vi "Decimate Segments.vi"(5 "Y Buffer":dbl[](array[numeric]), 6 "Swap Axes":bool, 7 "X Buffer":dbl[](array[numeric]), 8 "px Lengths":i32[](array[numeric]), 9 "px Starts":i32[](array[numeric]), 10 "Independent":dbl[](array[numeric]), 11 "Dependent":dbl[](array[numeric])) -> (2 "Decimated Data":cluster{"X":dbl[], "Y":dbl[]})   [LabVIEW 2020, in "VolatusGUIElements.lvlib"]
uses:
  VolatusGUIElements.lvlib
panel:
  out "Last X":dbl format="%<%H:%M:%S%1u>T"
  out "First X":dbl format="%<%H:%M:%S%1u>T"
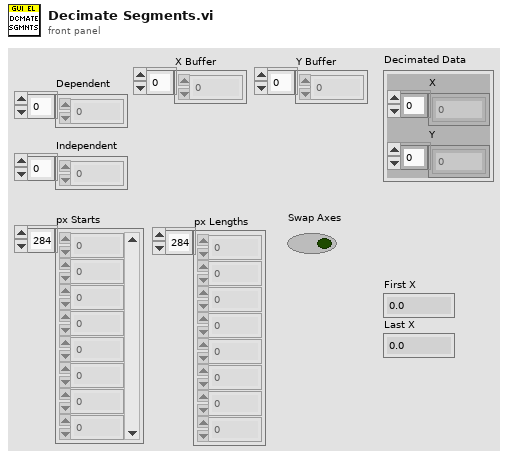
[diagram p1: front panel]
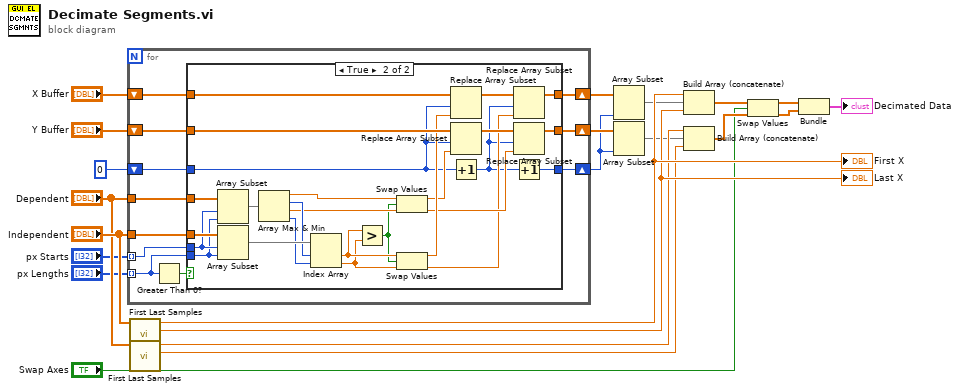
[diagram p0: block diagram]
diagram:
  n1 = for {
    shift-right: [w24] -> w11
    shift-left: "Y Buffer" -> [w27]
    shift-right: [w23] -> w12
    shift-left: "X Buffer" -> [w28]
    tunnel: "Independent" -> [w33]
    tunnel: "Dependent" -> [w32]
    tunnel: "px Starts" -> [w31] mode=indexing
    tunnel: "px Lengths" -> [w30] mode=indexing
    shift-right: [w25] -> w10
    shift-left: 0 -> [w26]
    n2 = Greater Than 0?(x=w30) -> (x > 0?=w29:bool)
    n3 = case shown="True" w29 {
      tunnel: w33 -> [_ w62]
      tunnel: w32 -> [_ w61]
      tunnel: w31 -> [_ w60]
      tunnel: w30 -> [_ w59]
      tunnel: w28 -> [w34 w49]
      tunnel: w27 -> [w35 w48]
      tunnel: w26 -> [w36 w45]
      tunnel: [w36 w39] -> w25
      tunnel: [w35 w38] -> w24
      tunnel: [w34 w37] -> w23
      frame False {
      }
      frame True {
        n4 = Array Subset(array=w61, index=w60, length=w59) -> (w58:dbl[])
        n5 = Array Subset(array=w62, index=w60, length=w59) -> (w57:dbl[])
        n6 = Array Max & Min(array=w58) -> (max value=w51:dbl, max index (indices)=w55:i32, min value=w52:dbl, min index (indices)=w56:i32)
        n7 = Index Array(array=w57, index #1=w55, index #2=w56) -> (element #1=w54:dbl, element #2=w53:dbl)
        n8 = Greater?(x=w54, y=w53) -> (0:w50:bool)
        n9 = Swap Values(12:w51, 13:w50, 14:w52) -> (1:w46:dbl, 3:w42:dbl)
        n10 = Swap Values(12:w54, 13:w50, 14:w53) -> (1:w47:dbl, 3:w41:dbl)
        n11 = Replace Array Subset(array=w49, new element=w47, index=w45) -> (w44:dbl[])
        n12 = Replace Array Subset(array=w48, new element=w46, index=w45) -> (w43:dbl[])
        n13 = Increment(x=w45) -> (x+1=w40:i32)
        n14 = Replace Array Subset(array=w44, new element=w41, index=w40) -> (w37:dbl[])
        n15 = Replace Array Subset(array=w43, new element=w42, index=w40) -> (w38:dbl[])
        n16 = Increment(x=w40) -> (x+1=w39:i32)
      }
    }
  }
  n17 = call "First Last Samples.vi"("Data"="Independent") -> ("Last"=w16:dbl, "First"=w17:dbl)  [unwired: 9 in]
  "First X" <- w17
  "Last X" <- w16
  n18 = call "First Last Samples.vi"("Data"="Dependent") -> ("Last"=w14:dbl, "First"=w15:dbl)  [unwired: 9 in]
  n19 = Array Subset(array=w12, length=w10) -> (w9:dbl[])  [unwired: 1 in]
  n20 = Array Subset(array=w11, length=w10) -> (w8:dbl[])  [unwired: 1 in]
  n21 = Build Array (concatenate)(w17, w9, w16) -> (w5:dbl[])
  n22 = Build Array (concatenate)(w15, w8, w14) -> (w4:dbl[])
  n23 = Swap Values(12:w5, 13:"Swap Axes", 14:w4) -> (1:w3:dbl[], 3:w2:dbl[])
  n24 = Bundle(w3, w2) -> (→"Decimated Data":cluster{dbl[], dbl[]})  [unwired: 1 in]
